vi "Calculate Next Generation.vi"(8 "error in":errorcluster, 10 "generation in":u32, 11 "cells in":bool[][](array[boolean])=[[FALSE, FALSE, TRUE, FALSE, FALSE, FALSE, FALSE, FALSE, FALSE, FALSE, FALSE, FALSE, FALSE, FALSE, FALSE, FALSE], [FALSE, FALSE, FALSE, TRUE, TRUE, FALSE, FALSE, FALSE, FALSE, FALSE, FALSE, FALSE, FALSE, FALSE, FALSE, FALSE], [FALSE, FALSE, FALSE, FALSE, FALSE, FALSE, FALSE, FALSE, FALSE, FALSE, FALSE, FALSE, FALSE, FALSE, FALSE, FALSE], [FALSE, FALSE, FALSE, FALSE, FALSE, FALSE, FALSE, FALSE, FALSE, FALSE, FALSE, FALSE, FALSE, FALSE, FALSE, FALSE], [FALSE, FALSE, FALSE, FALSE, FALSE, FALSE, FALSE, FALSE, FALSE, FALSE, FALSE, FALSE, FALSE, FALSE, FALSE, FALSE], [FALSE, FALSE, FALSE, FALSE, FALSE, FALSE, FALSE, FALSE, FALSE, FALSE, FALSE, FALSE, FALSE, FALSE, FALSE, FALSE], [FALSE, FALSE, FALSE, FALSE, FALSE, FALSE, FALSE, TRUE, FALSE, FALSE, FALSE, FALSE, FALSE, FALSE, FALSE, FALSE], [FALSE, FALSE, FALSE, FALSE, FALSE, FALSE, FALSE, FALSE, FALSE, FALSE, FALSE, FALSE, FALSE, FALSE, FALSE, FALSE], [FALSE, FALSE, FALSE, FALSE, FALSE, FALSE, FALSE, FALSE, FALSE, FALSE, FALSE, FALSE, FALSE, FALSE, FALSE, FALSE], [FALSE, FALSE, FALSE, FALSE, FALSE, FALSE, FALSE, FALSE, FALSE, FALSE, FALSE, FALSE, FALSE, TRUE, FALSE, FALSE], [FALSE, FALSE, FALSE, FALSE, FALSE, FALSE, FALSE, FALSE, FALSE, FALSE, FALSE, FALSE, TRUE, TRUE, FALSE, FALSE], [FALSE, FALSE, FALSE, FALSE, FALSE, FALSE, FALSE, FALSE, FALSE, FALSE, FALSE, FALSE, FALSE, FALSE, TRUE, FALSE], [FALSE, FALSE, FALSE, FALSE, FALSE, FALSE, FALSE, FALSE, FALSE, FALSE, FALSE, FALSE, FALSE, FALSE, FALSE, TRUE]]) -> (0 "error out":errorcluster, 1 "graph elements":T1, 2 "generation out":u32, 3 "cells out":bool[][](array[boolean])=[[FALSE, FALSE, FALSE, TRUE, FALSE, FALSE, FALSE, FALSE, FALSE, FALSE, FALSE, FALSE, FALSE, FALSE, FALSE, FALSE], [FALSE, FALSE, FALSE, TRUE, FALSE, FALSE, FALSE, FALSE, FALSE, FALSE, FALSE, FALSE, FALSE, FALSE, FALSE, FALSE], [FALSE, FALSE, FALSE, FALSE, FALSE, FALSE, FALSE, FALSE, FALSE, FALSE, FALSE, FALSE, FALSE, FALSE, FALSE, FALSE], [FALSE, FALSE, FALSE, FALSE, FALSE, FALSE, FALSE, FALSE, FALSE, FALSE, FALSE, FALSE, FALSE, FALSE, FALSE, FALSE], [FALSE, FALSE, FALSE, FALSE, FALSE, FALSE, FALSE, FALSE, FALSE, FALSE, FALSE, FALSE, FALSE, FALSE, FALSE, FALSE], [FALSE, FALSE, FALSE, FALSE, FALSE, FALSE, FALSE, FALSE, FALSE, FALSE, FALSE, FALSE, FALSE, FALSE, FALSE, FALSE], [FALSE, FALSE, FALSE, FALSE, FALSE, FALSE, FALSE, FALSE, FALSE, FALSE, FALSE, FALSE, FALSE, FALSE, FALSE, FALSE], [FALSE, FALSE, FALSE, FALSE, FALSE, FALSE, FALSE, FALSE, FALSE, FALSE, FALSE, FALSE, FALSE, FALSE, FALSE, FALSE], [FALSE, FALSE, FALSE, FALSE, FALSE, FALSE, FALSE, FALSE, FALSE, FALSE, FALSE, FALSE, FALSE, FALSE, FALSE, FALSE], [FALSE, FALSE, FALSE, FALSE, FALSE, FALSE, FALSE, FALSE, FALSE, FALSE, FALSE, FALSE, TRUE, TRUE, FALSE, FALSE], [FALSE, FALSE, FALSE, FALSE, FALSE, FALSE, FALSE, FALSE, FALSE, FALSE, FALSE, FALSE, TRUE, TRUE, TRUE, FALSE], [FALSE, FALSE, FALSE, FALSE, FALSE, FALSE, FALSE, FALSE, FALSE, FALSE, FALSE, FALSE, FALSE, TRUE, TRUE, FALSE], [FALSE, FALSE, FALSE, FALSE, FALSE, FALSE, FALSE, FALSE, FALSE, FALSE, FALSE, FALSE, FALSE, FALSE, FALSE, FALSE]], 4 "stop generation?":bool)   [LabVIEW 2021, in "Game of Life.lvlib"]
doc: "Any live cell with two or three live neighbors lives on to the next generation. Any dead cell with exactly three live neighbors becomes a live cell, as if by reproduction."
uses:
  Game of Life.lvlib
  Graph Elements.ctl
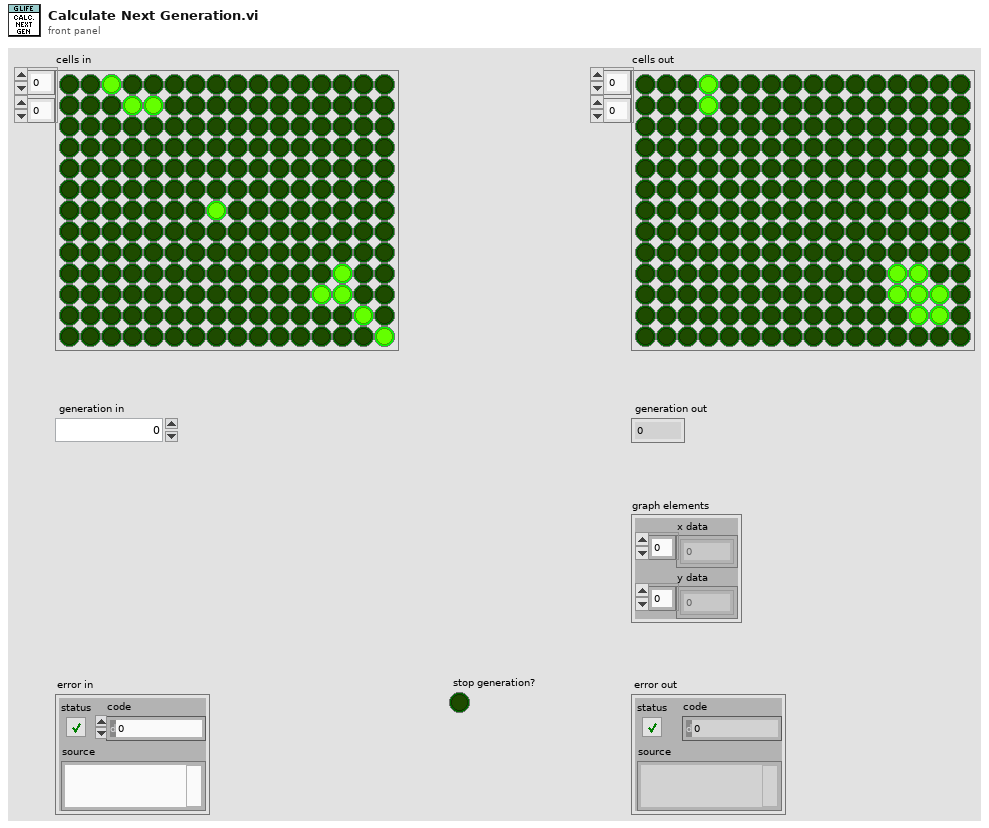
[diagram p1: front panel]
types:
  T1 = typedef "Game of Life.lvlib/Graph Elements.ctl" = cluster{"x data":dbl[], "y data":dbl[]}
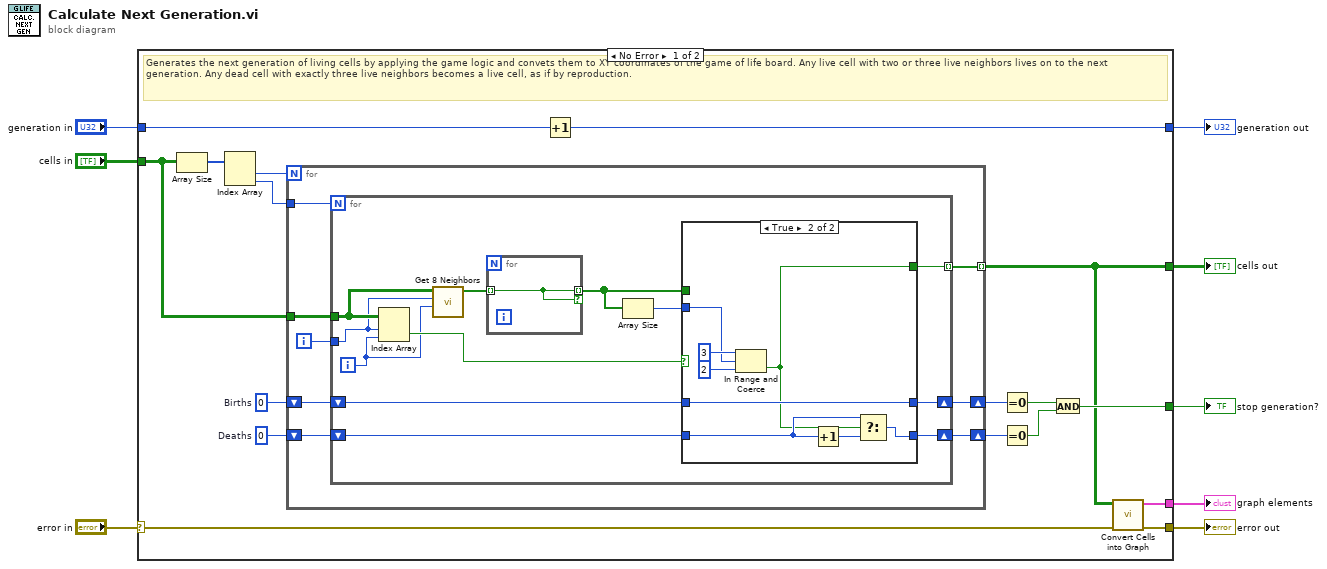
[diagram p0: block diagram]
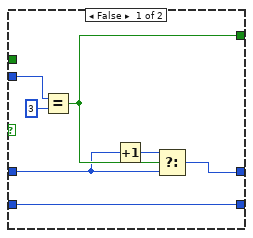
[diagram p2: hidden frame]
diagram:
  n1 = case shown="No Error" "error in" {
    selector: "error in" -> [w15 w64]
    tunnel: "cells in" -> [w20 w63]
    tunnel: [w10 w63] -> w7
    tunnel: [w14 w64] -> w6
    tunnel: "generation in" -> [w19 w62]
    tunnel: [w18 w62] -> w4
    tunnel: [w11 _] -> w2
    tunnel: [w9 _] -> w1
    frame No Error {
      w21 = 0  # Deaths
      w22 = 0  # Births
      # "Generates the next generation of living cells by applying the game logic and convets them to XY coordinates of the game of life board. Any live cell with two or three live neighbors lives on to the next generation. Any dead cell with exactly three live neighbors becomes a live cell, as if by reproduction."
      n2 = Array Size(array=w20) -> (size(s)=w25:i32[])
      n3 = Index Array(array=w25) -> (element #1=w24:i32, element #2=w23:i32)  [unwired: 2 in]
      n4 = for {
        N: w24 -> [_]
        tunnel: w23 -> [w32]
        shift-right: [w28] -> w13
        shift-left: w22 -> [w31]
        shift-right: [w27] -> w12
        shift-left: w21 -> [w30]
        tunnel: w20 -> [w29]
        tunnel: [w26] -> w10 mode=indexing
        i -> [w33]
        n5 = for {
          N: w32 -> [_]
          tunnel: w33 -> [w38]
          tunnel: [w45] -> w26 mode=indexing
          shift-right: [w44] -> w28
          shift-left: w31 -> [w43]
          shift-right: [w41] -> w27
          shift-left: w30 -> [w42]
          tunnel: w29 -> [w39]
          i -> [w37]
          n6 = Index Array(array=w39, index (row)=w38, index (col)=w37) -> (element=w40:bool)
          n7 = call "Get 8 Neighbors.vi"("column"=w37, "row"=w38, "cells in"=w39) -> ("cells living"=w36:bool[])  [unwired: 8 in]
          n8 = for {
            tunnel: w36 -> [w46] mode=indexing
            tunnel: [w46] -> w34 mode=indexing if=w46
          }
          n9 = Array Size(array=w34) -> (size(s)=w35:i32)
          n10 = case shown="True" w40 {
            tunnel: [w51 w55] -> w45
            tunnel: [w48 w59] -> w44
            tunnel: w43 -> [w47 w59]
            tunnel: w42 -> [w49 w57]
            tunnel: [w49 w54] -> w41
            tunnel: w35 -> [w52 w58]
            tunnel: w34 -> [_ _]
            frame False {
              n11 = Equal?(x=w52, y=3) -> (x = y?=w51:bool)
              n12 = Increment(x=w47) -> (x+1=w50:i32)
              n13 = Select(t=w50, s=w51, f=w47) -> (s? t:f=w48:i32)
            }
            frame True {
              n14 = In Range and Coerce(upper limit=3, x=w58, lower limit=2) -> (In Range?=w55:bool)  [unwired: 1 out]
              n15 = Increment(x=w57) -> (x+1=w56:i32)
              n16 = Select(t=w57, s=w55, f=w56) -> (s? t:f=w54:i32)
            }
          }
        }
      }
      n17 = Increment(x=w19) -> (x+1=w18:u32)
      n18 = Equal To 0?(x=w13) -> (x = 0?=w16:bool)
      n19 = Equal To 0?(x=w12) -> (x = 0?=w17:bool)
      n20 = And(x=w16, y=w17) -> (x .and. y?=w11:bool)
      n21 = call "Convert Cells into Graph.vi"("error in"=w15, "cells in"=w10) -> ("error out"=w14:errorcluster, "graph elements"=w9:T1)  [unwired: 8 in]
    }
    frame Error {
    }
  }
  "cells out" <- w7
  "error out" <- w6
  "generation out" <- w4
  "stop generation?" <- w2
  "graph elements" <- w1
